vi "Base64 Conversion.vi"(11 "String":string) -> (3 "Base64 String":string)   [LabVIEW 2011, in "i3-oauth.lvlib"]
uses:
  i3-oauth.lvlib
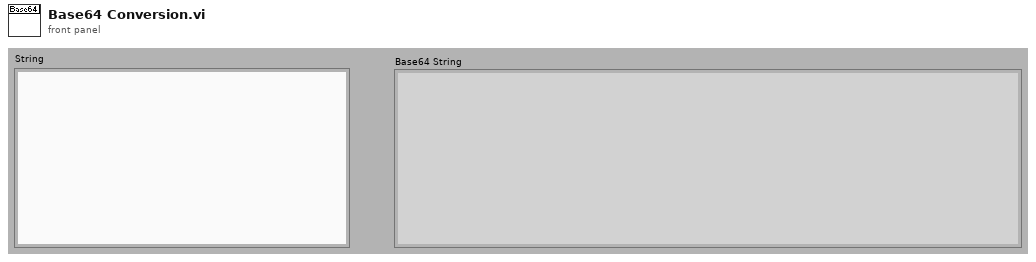
[diagram p1: front panel]
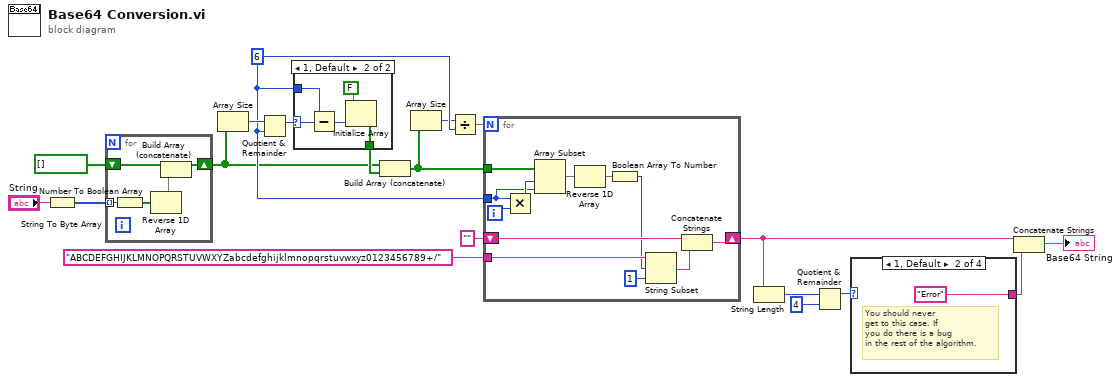
[diagram p0: block diagram]
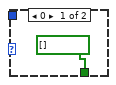
[diagram p2: hidden frame]
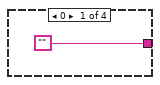
[diagram p3: hidden frame]
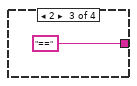
[diagram p4: hidden frame]
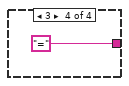
[diagram p5: hidden frame]
diagram:
  w4 = 6 ("y")
  n1 = String To Byte Array(string="String") -> (unsigned byte array=w18:u8[])
  n2 = for {
    tunnel: w18 -> [w24] mode=indexing
    shift-right: [w21] -> w3
    shift-left: bool[] [] -> [w23]
    n3 = Number To Boolean Array(number=w24) -> (Boolean array=w22:bool[])
    n4 = Reverse 1D Array(array=w22) -> (reversed array=w20:bool[])
    n5 = Build Array (concatenate)(w23, w20) -> (w21:bool[])
  }
  n6 = Array Size(array=w3) -> (size(s)=w7:i32)
  n7 = Quotient & Remainder(x=w7, y=w4) -> (x-y*floor(x/y)=w6:i32)  [unwired: 1 out]
  n8 = case shown="1, Default" w6 {
    selector: w6 -> [_ w29]
    tunnel: [bool[] [] w26] -> w5
    tunnel: w4 -> [_ w28]
    frame 0 {
    }
    frame 1, Default {
      n9 = Subtract(x=w28, y=w29) -> (x-y=w30:i32)
      n10 = Initialize Array(FALSE, w30) -> (w26:bool[])
    }
  }
  n11 = Build Array (concatenate)(w3, w5) -> (w2:bool[])
  n12 = Array Size(array=w2) -> (size(s)=w1:i32)
  n13 = Divide(x=w1, y=w4) -> (x/y=w8:dbl)
  n14 = for {
    N: w8 -> [_]
    tunnel: w2 -> [w41]
    tunnel: w4 -> [w39]
    tunnel: "ABCDEFGHIJKLMNOPQRSTUVWXYZabcdefghijklmnopqrstuvwxyz0123456789+/" -> [w38]
    shift-right: [w36] -> w10
    shift-left: "" -> [w35]
    i -> [w42]
    n15 = Multiply(x=w39, y=w42) -> (x*y=w40:i32)
    n16 = Array Subset(array=w41, index=w40, length=w39) -> (w31:bool[])
    n17 = Reverse 1D Array(array=w31) -> (reversed array=w32:bool[])
    n18 = Boolean Array To Number(Boolean array=w32) -> (number=w33:u32)
    n19 = String Subset(string=w38, offset (0)=w33, length (rest)=1 ("length (rest)")) -> (substring=w34:string)
    n20 = Concatenate Strings(w35, w34) -> (w36:string)
  }
  n21 = String Length(string=w10) -> (length=w14:i32)
  n22 = Quotient & Remainder(x=w14, y=4) -> (x-y*floor(x/y)=w12:i32)  [unwired: 1 out]
  n23 = case shown="1, Default" w12 {
    tunnel: ["" "Error" "==" "="] -> w11
    frame 0 {
    }
    frame 1, Default {
      # "You should never\nget to this case. If\nyou do there is a bug\nin the rest of the algorithm."
    }
    frame 2 {
    }
    frame 3 {
    }
  }
  n24 = Concatenate Strings(w10, w11) -> (→"Base64 String":string)
